vi "st_str RealiseArrayData(ViForIzm).vi"(8 "error in (no error)":errorcluster, 11 "AllParametrArray":dbl[][](array[numeric])) -> (0 "error out":errorcluster, 2 "appended array":cluster{dbl[], dbl[]}[](array[cluster]), 3 "Graph Data":waveform(dbl)[](array[waveform]))   [LabVIEW 2017]
doc: "Generates sample waveforms according to the signal type in the HW Config input."
panel:
  out "XY Graph":cluster{dbl[], dbl[]}(graph)
  # "Ku"
  # "f"
  # "b"
  # "a"
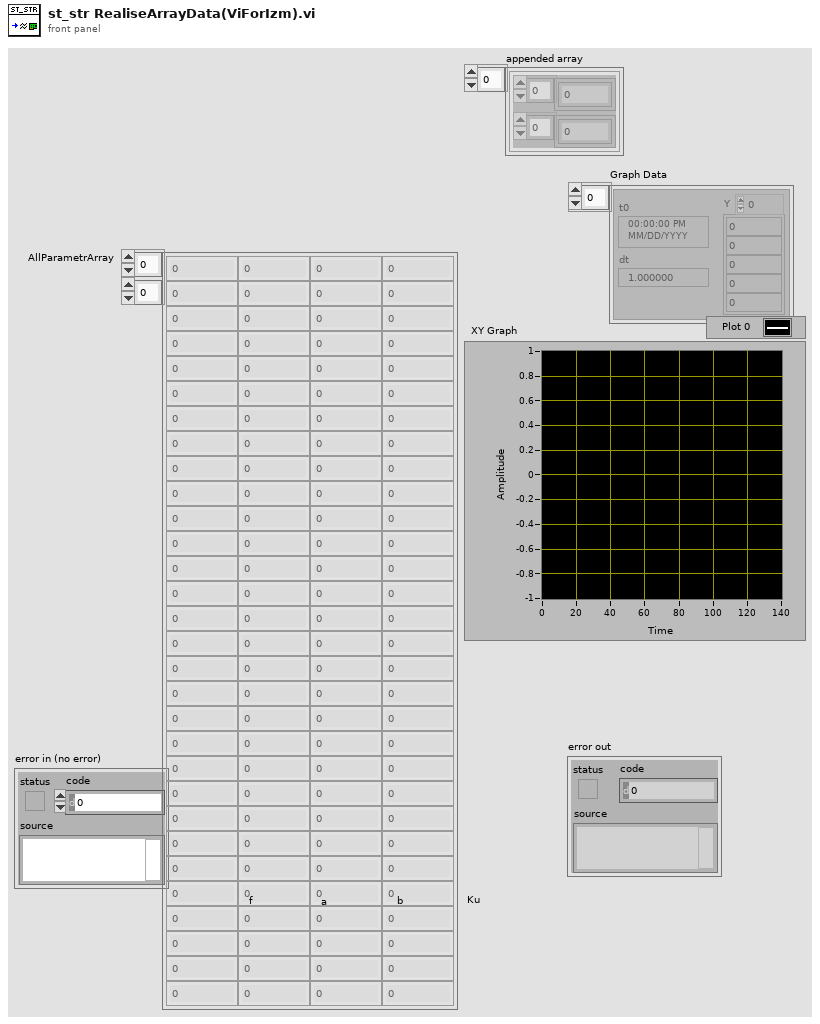
[diagram p1: front panel]
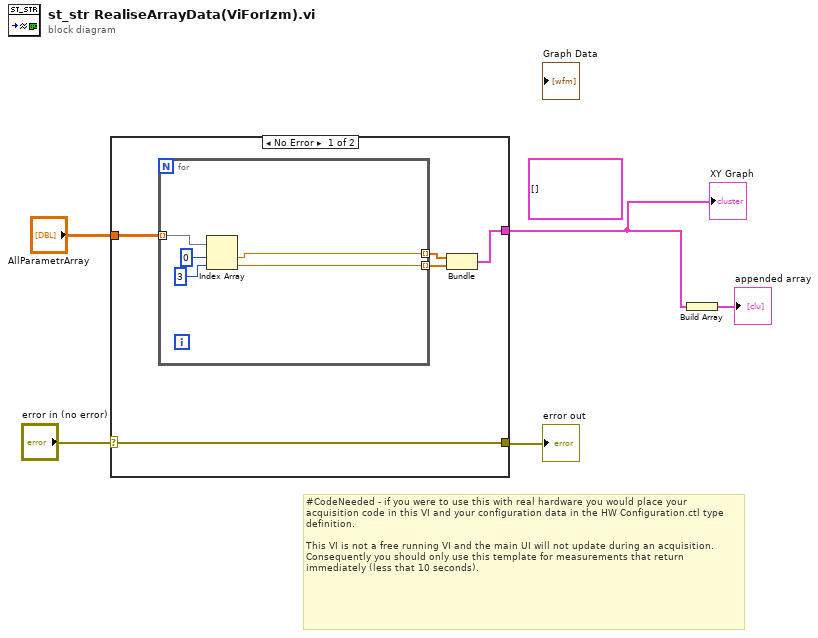
[diagram p0: block diagram]
diagram:
  (unwired) cluster{"X":dbl[], "Y":dbl[]}[] [] ("XY graph 2")
  # "#CodeNeeded - if you were to use this with real hardware you would place your acquisition code in this VI and your configuration data in the HW Configuration.ctl type definition.\n\nThis VI is not a free running VI and the main UI will not update during an acquisition.  Consequently you should only use this template for measurements that return immediately (less that 10 seconds)."
  n1 = case shown="No Error" "error in (no error)" {
    selector: "error in (no error)" -> [w10 w16]
    tunnel: [w10 w16] -> w4
    tunnel: "AllParametrArray" -> [w9 _]
    tunnel: [w8 _] -> w1
    frame No Error {
      n2 = for {
        tunnel: w9 -> [w15] mode=indexing
        tunnel: [w12] -> w7 mode=indexing
        tunnel: [w11] -> w6 mode=indexing
        n3 = Index Array(array=w15, index #1=0 ("index"), index #2=3 ("index")) -> (element #1=w12:dbl, element #2=w11:dbl)
      }
      n4 = Bundle(w7, w6) -> (w8:cluster{dbl[], dbl[]})  [unwired: 1 in]
    }
    frame Error {
    }
  }
  "error out" <- w4
  "XY Graph" <- w1
  n5 = Build Array(w1) -> (→"appended array":cluster{dbl[], dbl[]}[])
